vi "AudioFileCompleteBroadcast_Parse.vi"(8 "error in (no error)":errorcluster, 11 "message":variant) -> (0 "error out":errorcluster, 2 "data":T1)   [LabVIEW 2017, in "EmsaAudio.lvlib"]
uses:
  <vilib>/addons/InsightCM/Devices/Shared/Emsa/EmsaAudio/EmsaAudio.lvlib
  <vilib>/addons/InsightCM/Devices/Shared/Emsa/EmsaAudio/controls/AudioFileCompleteBroadcast.ctl
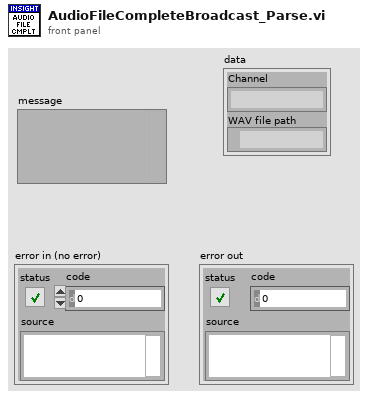
[diagram p1: front panel]
types:
  T1 = typedef "EmsaAudio.lvlib/AudioFileCompleteBroadcast.ctl" = cluster{"Channel":string, "WAV file path":path}
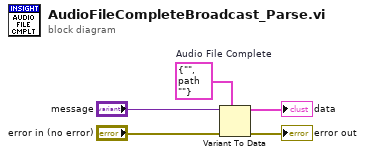
[diagram p0: block diagram]
diagram:
  w2 = T1 {"Channel"="", "WAV file path"=path ""}  # Audio File Complete
  n1 = Variant To Data(error in="error in (no error)", type=w2, Variant="message") -> (data=→"data":T1, error out=→"error out":errorcluster)
